vi "Goto.vi"(6 "Home?":bool, 7 "Speed":i32, 8 "error in (no error)":errorcluster, 9 "channel":i32(ring)=1 items=["Channel1"=1, "Channel2"=2, "Channel3"=3, "Channel4"=4], 10 "New Position":sgl, 11 "TranslationStage in":refnum<class "TranslationStagesInterface.lvclass">) -> (0 "error out":errorcluster, 3 "TranslationStage out":refnum<class "TranslationStagesInterface.lvclass">)   [LabVIEW 2023, in "TranslationStage Library.lvlib" / "TranslationStage.lvlib" / "TranslationStagesInterface.lvclass"]
uses:
  TranslationStagesInterface.lvclass
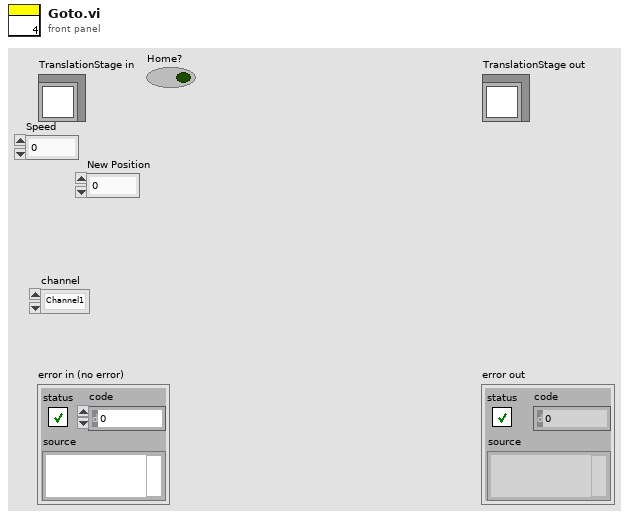
[diagram p1: front panel]
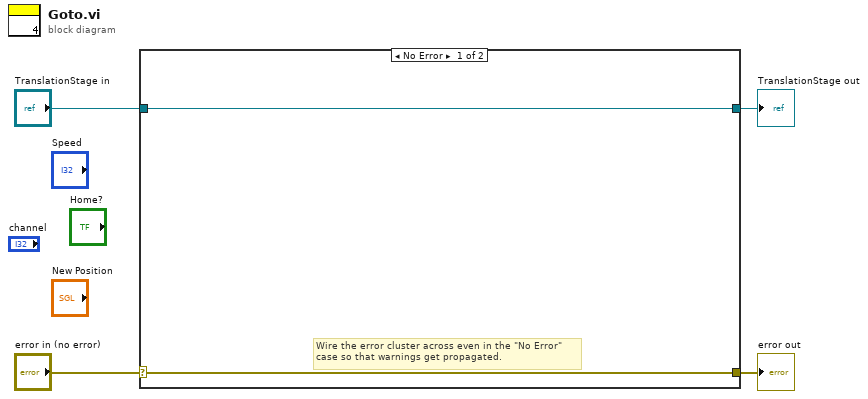
[diagram p0: block diagram]
diagram:
  n1 = case shown="No Error" "error in (no error)" {
    selector: "error in (no error)" -> [w5 w8]
    tunnel: [w5 w8] -> w3
    tunnel: [w6 w7] -> w1
    tunnel: "TranslationStage in" -> [w6 w7]
    frame No Error {
      # "Wire the error cluster across even in the \"No Error\"\ncase so that warnings get propagated."
    }
    frame Error {
    }
  }
  "error out" <- w3
  "TranslationStage out" <- w1
